vi "RM.internalAPITests.vi"() -> ()   [LabVIEW 2016, in "FPGA Addon Shared.lvlib"]
uses:
  FPGA Addon Shared.lvlib
  RM.resourceDirection.ctl
  RM.resourceType.ctl
panel:
  out "reservers":string[](array[string])
  out "names in bitfile":string[](array[string])
  out "found? 4":bool
  out "replaced 2":bool
  out "found? 3":bool
  out "found? 2":bool
  out "reservation DB out":variant
  out "found?":bool
  out "error out":errorcluster
  out "replaced":bool
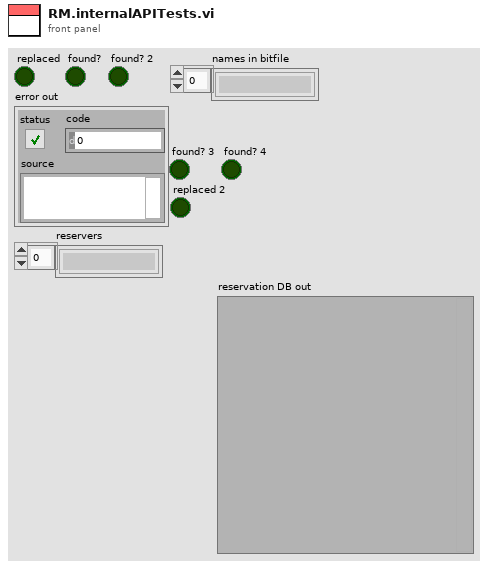
[diagram p1: front panel]
types:
  T1 = typedef "FPGA Addon Shared.lvlib/RM.resourceType.ctl" = enum16{"Scalar", "Waveform"}
  T2 = typedef "FPGA Addon Shared.lvlib/RM.resourceDirection.ctl" = enum16{"To FPGA", "From FPGA"}
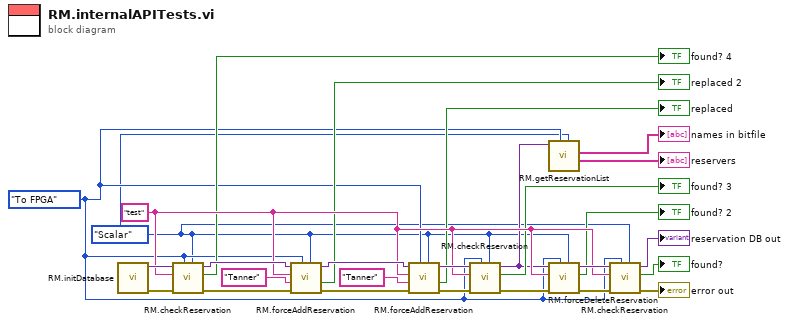
[diagram p0: block diagram]
diagram:
  w1 = RM.resourceType."Scalar" ("Resource Type")
  w2 = RM.resourceDirection."To FPGA" ("Direction")
  w15 = "test" ("name in bitfile")
  n1 = call "RM.initDatabase.vi"() -> ("error out"=w26:errorcluster, "variant out"=w27:variant)  [unwired: 10 in]
  n2 = call "RM.checkReservation.vi"("Resource Type"=w1, "Direction"=w2, "error in"=w26, "name in bitfile"=w15, "reservation DB in"=w27) -> ("error out"=w24:errorcluster, "found?"=→"found? 4":bool, "reservation DB out"=w25:variant)  [unwired: 4 in]
  n3 = call "RM.forceAddReservation.vi"("Resource Type"=w1, "Direction"=w2, "error in"=w24, "reserver"="Tanner", "name in bitfile"=w15, "reservation DB in"=w25) -> ("error out"=w23:errorcluster, "replaced"=→"replaced 2":bool, "reservation DB out"=w18:variant)  [unwired: 3 in]
  n4 = call "RM.forceAddReservation.vi"("Resource Type"=w1, "Direction"=w2, "error in"=w23, "reserver"="Tanner", "name in bitfile"=w15, "reservation DB in"=w18) -> ("error out"=w19:errorcluster, "replaced"=→"replaced":bool, "reservation DB out"=w17:variant)  [unwired: 3 in]
  n5 = call "RM.checkReservation.vi"("Resource Type"=w1, "Direction"=w2, "error in"=w19, "name in bitfile"=w15, "reservation DB in"=w17) -> ("error out"=w22:errorcluster, "found?"=→"found? 3":bool, "reservation DB out"=w5:variant)  [unwired: 4 in]
  n6 = call "RM.getReservationList.vi"("Resource Type"=w1, "Direction"=w2, "reservation DB in"=w5) -> ("reservers"=→"reservers":string[], "names in bitfile"=→"names in bitfile":string[])  [unwired: 5 in, 2 out]
  n7 = call "RM.forceDeleteReservation.vi"("Resource Type"=w1, "Direction"=w2, "error in"=w22, "name in bitfile"=w15, "reservation DB in"=w5) -> ("error out"=w20:errorcluster, "found?"=→"found? 2":bool, "reservation DB out"=w21:variant)  [unwired: 4 in]
  n8 = call "RM.checkReservation.vi"("Resource Type"=w1, "Direction"=w2, "error in"=w20, "name in bitfile"=w15, "reservation DB in"=w21) -> ("error out"=→"error out":errorcluster, "found?"=→"found?":bool, "reservation DB out"=→"reservation DB out":variant)  [unwired: 4 in]
